vi "Read Instrument type.vi"(8 "error in (no error)":errorcluster, 11 "InstControl in":refnum<class "InstrControl.lvclass">) -> (0 "error out":errorcluster, 2 "Instrument type":u16(ring) items=["Supply", "LCR"], 3 "InstControl out":refnum<class "InstrControl.lvclass">)   [LabVIEW 2018, in "InstrControl.lvclass"]
uses:
  InstrControl.lvclass
  InstrControl.lvclass/InstrControl.ctl
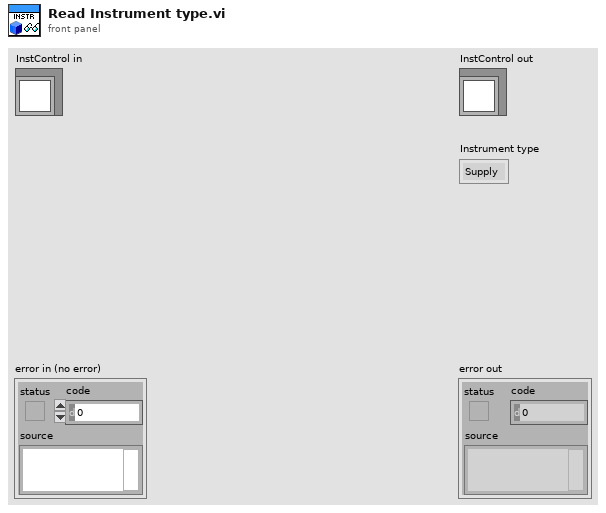
[diagram p1: front panel]
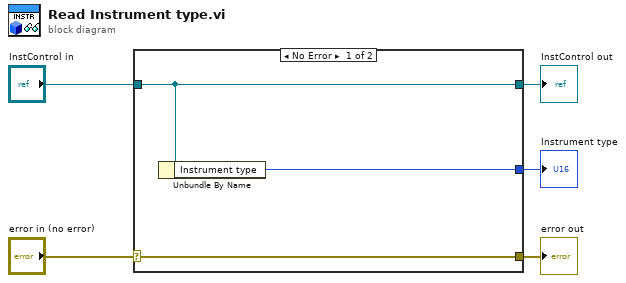
[diagram p0: block diagram]
diagram:
  n1 = case shown="No Error" "error in (no error)" {
    selector: "error in (no error)" -> [w8 w9]
    tunnel: [w8 w9] -> w4
    tunnel: [w7 w10] -> w2
    tunnel: "InstControl in" -> [w7 w10]
    tunnel: [w6 _] -> w1
    frame No Error {
      n2 = Unbundle By Name(w7) -> ("Instrument type"=w6:u16)
    }
    frame Error {
    }
  }
  "error out" <- w4
  "InstControl out" <- w2
  "Instrument type" <- w1
